vi "benchmarks_fileMD5.vi"() -> ()   [LabVIEW 2013]
uses:
  MD5/MD5.lvclass
  MD5/Enqueue File.vi
  MD5/MD5.lvlib
panel:
  out "% gain":dbl
  out "LVOS":string
  out "NI":string
  out "LVOS":dbl
  out "NI":dbl
  in  "filepath":path
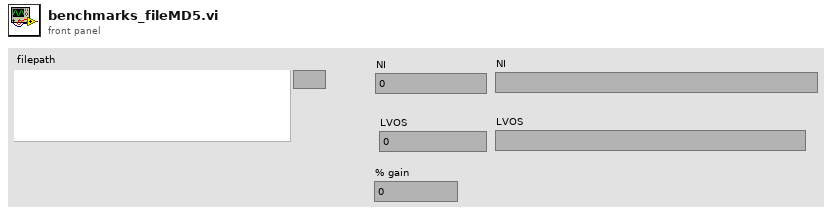
[diagram p1: front panel]
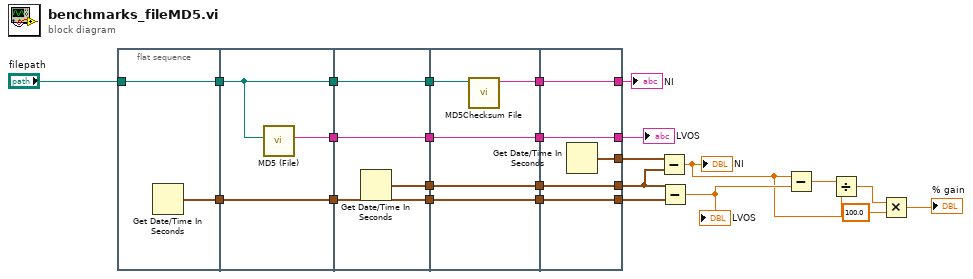
[diagram p0: block diagram]
diagram:
  n1 = flat-sequence {
    tunnel: "filepath" -> [w27]
    tunnel: [w27] -> w22
    tunnel: [w26] -> w21
    tunnel: [w30] -> w24
    tunnel: w22 -> [w30]
    tunnel: w21 -> [w29]
    tunnel: [w29] -> w16
    tunnel: [w28] -> w9
    tunnel: w24 -> [w34]
    tunnel: [w34] -> w23
    tunnel: [w33] -> w19
    tunnel: [w32] -> w17
    tunnel: w16 -> [w32]
    tunnel: [w31] -> w10
    tunnel: w9 -> [w31]
    tunnel: w23 -> [w39]
    tunnel: [w38] -> w20
    tunnel: w19 -> [w38]
    tunnel: [w37] -> w18
    tunnel: w17 -> [w37]
    tunnel: [w36] -> w12
    tunnel: [w35] -> w11
    tunnel: w10 -> [w35]
    tunnel: [w44] -> w14
    tunnel: w20 -> [w44]
    tunnel: [w43] -> w13
    tunnel: w18 -> [w43]
    tunnel: [w42] -> w15
    tunnel: [w41] -> w8
    tunnel: w12 -> [w41]
    tunnel: [w40] -> w7
    tunnel: w11 -> [w40]
    frame #0 {
      n2 = Get Date/Time In Seconds() -> (seconds since 1Jan1904=w26:timestamp)
    }
    frame #1 {
      n3 = call "MD5 (File).vi"("filepath"=w30) -> ("MD5 hash"=w28:string)  [unwired: 10 in]
    }
    frame #2 {
      n4 = Get Date/Time In Seconds() -> (seconds since 1Jan1904=w33:timestamp)
    }
    frame #3 {
      n5 = call <vilib>:"MD5Checksum File.vi"("Path"=w39) -> ("MD5 message-digest"=w36:string)  [unwired: 9 in, 1 out]
    }
    frame #4 {
      n6 = Get Date/Time In Seconds() -> (seconds since 1Jan1904=w42:timestamp)
    }
  }
  n7 = Subtract(x=w15, y=w14) -> (x-y=w1:dbl)
  "NI" <- w1
  n8 = Subtract(x=w14, y=w13) -> (x-y=w6:dbl)
  "LVOS" <- w6
  n9 = Subtract(x=w1, y=w6) -> (x-y=w5:dbl)
  n10 = Divide(x=w5, y=w1) -> (x/y=w3:dbl)
  n11 = Multiply(x=w3, y=100.0) -> (x*y=→"% gain":dbl)
  "NI" <- w8
  "LVOS" <- w7
